vi "Write All Pulse.vi"(8 "error in":errorcluster, 10 "Trigger Settings All":T1 {"Delay" format="%#_g s"; "Interval" format="%#_g s"; "Width" format="%#_g s"}, 11 "Electronic Load in":refnum<class "Electronic Load.lvclass">) -> (0 "error out":errorcluster, 3 "Electronic Load out":refnum<class "Electronic Load.lvclass">)   [LabVIEW 2019, in "Electronic Load.lvlib" / "Electronic Load.lvclass"]
uses:
  Library/Electronic Load.lvclass
  C:/Users/Public/Documents/Development/builds/Instruments/Instruments.lvlibp/Library/Instruments.lvclass
  Custom Controls/Trigger Settings.ctl
  Custom Controls/E-Load Mode.ctl
  Library/Electronic Load.lvclass/Electronic Load.ctl
  builds/Instruments/Instruments.lvlibp/Private/Polymorphic/Special/Event from String.vi
  builds/Instruments/Instruments.lvlibp/Accessors/Command with Logging.vi
  builds/Instruments/Instruments.lvlibp/Library/Instruments.lvclass
  builds/Instruments/Instruments.lvlibp
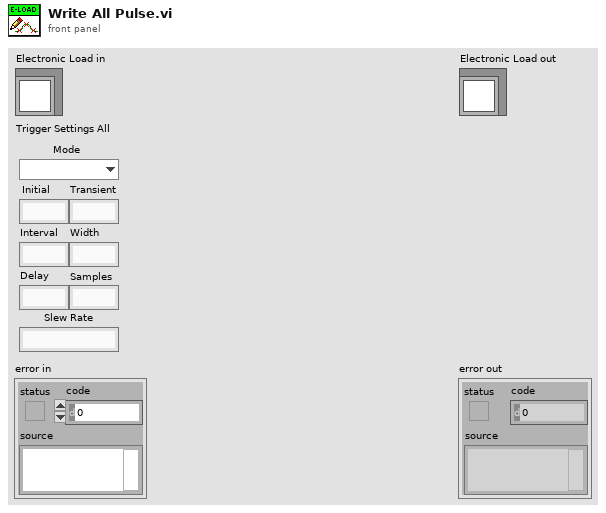
[diagram p1: front panel]
types:
  T1 = typedef "Electronic Load.lvlib/Electronic Load.lvclass/Trigger Settings.ctl" = cluster{"Mode":T2, "Initial":dbl, "Transient":dbl, "Interval":dbl, "Width":dbl, "Delay":dbl, "Data Pts":i32, "Slew Rate":dbl}
  T2 = typedef "Electronic Load.lvlib/Electronic Load.lvclass/E-Load Mode.ctl" = enum16{"Current", "Resistance", "Voltage"}
  T3 = cluster{"Timestamp":timestamp, "Description":string, "Data":string}
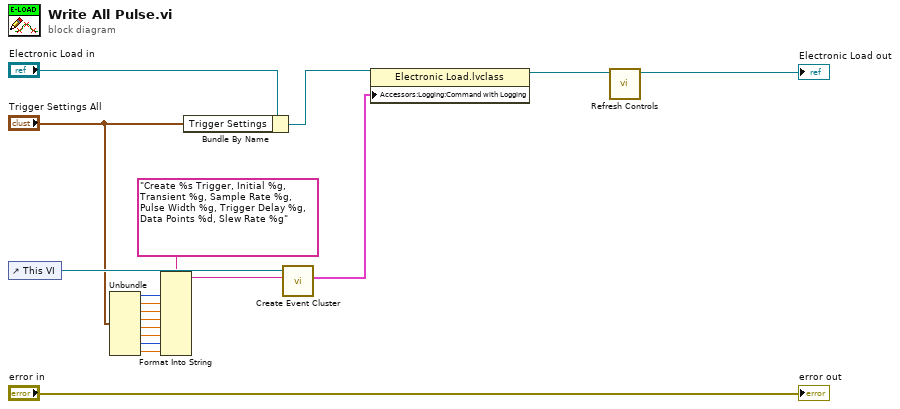
[diagram p0: block diagram]
diagram:
  n1 = control-ref of="This VI"() -> (w8:refnum<vi>)
  n2 = Unbundle("Trigger Settings All") -> ("Mode"=w16:T2, "Initial"=w15:dbl, "Transient"=w14:dbl, "Interval"=w13:dbl, "Width"=w12:dbl, "Delay"=w11:dbl, "Data Pts"=w10:i32, "Slew Rate"=w9:dbl)
  n3 = Format Into String(format string="Create %s Trigger, Initial %g, Transient %g, Sample Rate %g,  Pulse Width %g, Trigger Delay %g, Data Points %d, Slew Rate %g", w16, w15, w14, w13, w12, w11, w10, w9) -> (resulting string=w7:string)  [unwired: 2 in, 1 out]
  n4 = Bundle By Name(cluster="Electronic Load in", "Trigger Settings"="Trigger Settings All") -> (w6:refnum<class "Electronic Load.lvclass">)
  n5 = call-poly "Create Event Cluster.vi"("Value"=w7, "VI Refnum"=w8) -> ("Event Data"=w5:T3)  [unwired: 9 in]
  n6 = property class="Electronic Load.lvclass"(reference=w6, "Accessors:Logging:Command with Logging"=w5) -> (reference out=w2:refnum<class "Electronic Load.lvclass">)  [unwired: 1 in, 1 out]
  n7 = call "Refresh Controls.vi"("Electronic Load in"=w2) -> ("Electronic Load out"=→"Electronic Load out":refnum<class "Electronic Load.lvclass">)  [unwired: 9 in, 1 out]
  "error out" <- "error in"
